vi "Release Email Ref.vi"(8 "error in (no error)":errorcluster, 11 "StmpEmail in":refnum<class "StmpEmail.lvclass">) -> (0 "error out":errorcluster, 3 "StmpEmail out":refnum<class "StmpEmail.lvclass">)   [LabVIEW 2015, in "StmpEmail.lvclass"]
uses:
  StmpEmail.lvclass
  StmpEmail.lvclass/StmpEmail.ctl
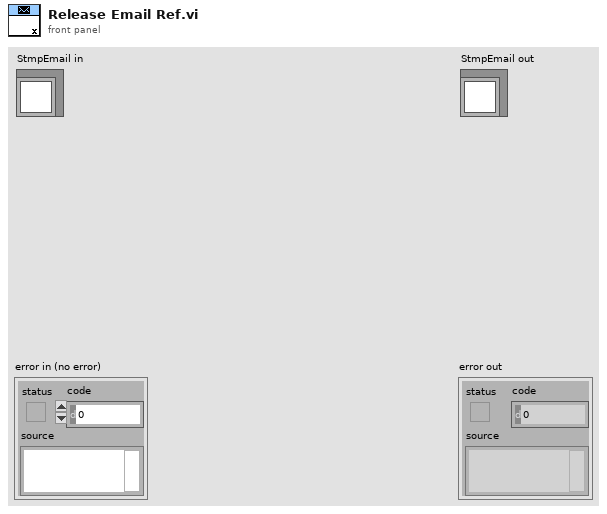
[diagram p1: front panel]
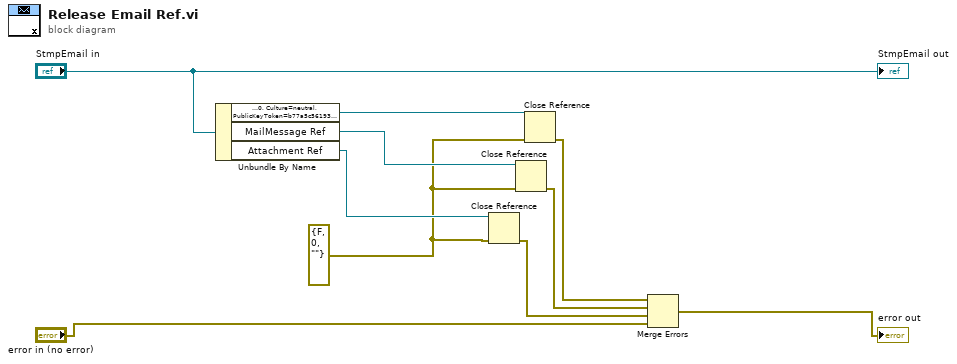
[diagram p0: block diagram]
diagram:
  w6 = errorcluster {"status"=FALSE, "code"=0, "source"=""} ("error constant")
  n1 = Unbundle By Name("StmpEmail in") -> ("SmtpEamil Ref"=w9:refnum<k24>, "MailMessage Ref"=w8:refnum<k24>, "Attachment Ref"=w7:refnum<k24>)
  n2 = Close Reference(reference=w7, error in (no error)=w6) -> (error out=w3:errorcluster)
  n3 = Close Reference(reference=w8, error in (no error)=w6) -> (error out=w4:errorcluster)
  n4 = Close Reference(reference=w9, error in (no error)=w6) -> (error out=w5:errorcluster)
  n5 = Merge Errors(w5, w4, w3, "error in (no error)") -> (→"error out":errorcluster)
  "StmpEmail out" <- "StmpEmail in"
